vi "Do Request.vi"(7 "Processing In":refnum<class "Processing.lvclass">, 11 "HTTPCmdController in":refnum<class "HTTPCmdController.lvclass">) -> (0 "error out":errorcluster, 5 "Processing":refnum<class "Processing.lvclass">)   [LabVIEW 2020, in "Volatus.lvlib" / "HTTPCmdController.lvclass"]
doc: "A controller's main job is to respond to a request by generating a response. The response value must be specified by calling Set Response.vi on the Processing class that's passed through the VI otherwise an error will be generated.\n\nThere are several helpers available for common response types:\nGenerating HTML content programmatically - Create Basic Response.vi\nStreaming a file from disk - Create File Response.vi\nRedirecting the user to another URL - Create Redirect Response.vi\n\nFile responses are streamed in chunks and do not load the entire file into memory at once to send in the response which allows serving large files more efficiently."
uses:
  HTTPCmdController.lvclass
  lv-http-server/HTTP Server/Processing/Processing.lvclass
  HTTPCmdController.lvclass/HTTPCmdController.ctl
  Http Cmd Type.ctl
  Volatus.lvlib
  Http Chan Cmd.ctl
  MessageQ/MessageQ.lvclass
  lv-http-util/HTTP Utils/Response/Response.lvclass
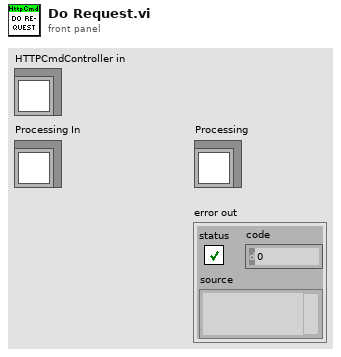
[diagram p1: front panel]
types:
  T1 = typedef "Volatus.lvlib/Http Chan Cmd.ctl" = cluster{"Type":T2, "Channel":string, "Value":dbl}
  T2 = typedef "Volatus.lvlib/Http Cmd Type.ctl" = enum16{"Digital", "Numeric"}
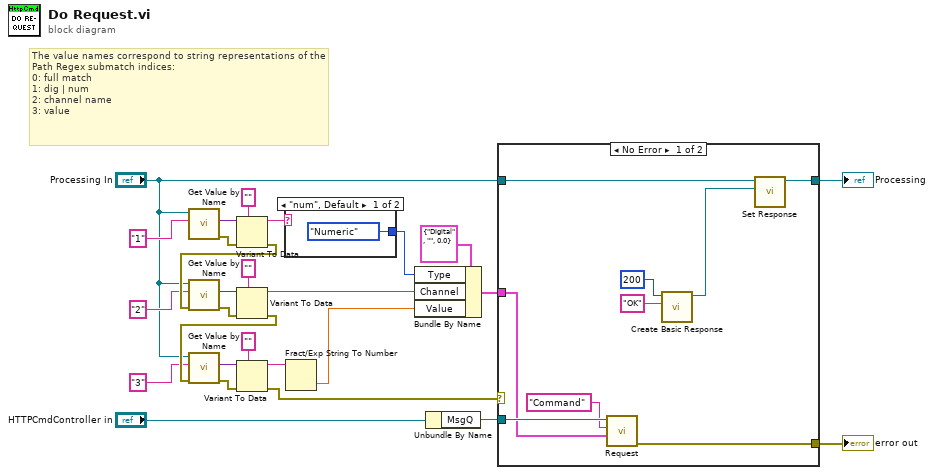
[diagram p0: block diagram]
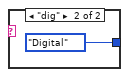
[diagram p3: hidden frame]
diagram:
  # "The value names correspond to string representations of the Path Regex submatch indices:\n0: full match\n1: dig | num\n2: channel name\n3: value"
  n1 = call "Get Value by Name.vi"("Name"="1", "Processing in"="Processing In") -> ("error out"=w10:errorcluster, "Value"=w24:variant)  [unwired: 7 in, 1 out]
  n2 = Variant To Data(error in=w10, type="", Variant=w24) -> (data=w14:string, error out=w27:errorcluster)
  n3 = call "Get Value by Name.vi"("error in (no error)"=w27, "Name"="2", "Processing in"="Processing In") -> ("error out"=w9:errorcluster, "Value"=w21:variant)  [unwired: 6 in, 1 out]
  n4 = Variant To Data(error in=w9, type="", Variant=w21) -> (data=w12:string, error out=w26:errorcluster)
  n5 = call "Get Value by Name.vi"("error in (no error)"=w26, "Name"="3", "Processing in"="Processing In") -> ("error out"=w8:errorcluster, "Value"=w18:variant)  [unwired: 6 in, 1 out]
  n6 = Variant To Data(error in=w8, type="", Variant=w18) -> (data=w16:string, error out=w5:errorcluster)
  n7 = case shown="\"num\", Default" w14 {
    tunnel: [Http_Cmd_Type."Numeric" ("Type") Http_Cmd_Type."Digital" ("Type")] -> w13
    frame "num", Default {
    }
    frame "dig" {
    }
  }
  n8 = Fract/Exp String To Number(string=w16) -> (number=w11:dbl)  [unwired: 3 in, 1 out]
  n9 = Bundle By Name(cluster=T1 {"Type"=enum."Digital", "Channel"="", "Value"=0.0} ("Http Chan Cmd"), "Type"=w13, "Channel"=w12, "Value"=w11) -> (w3:T1)
  n10 = Unbundle By Name("HTTPCmdController in") -> ("MsgQ"=w4:refnum<class "MessageQ.lvclass">)
  n11 = case shown="No Error" w5 {
    selector: w5 -> [_ w39]
    tunnel: "Processing In" -> [w34 w40]
    tunnel: w4 -> [w38 _]
    tunnel: w3 -> [w36 _]
    tunnel: [w35 w39] -> w2
    tunnel: [w31 w40] -> w1
    frame No Error {
      n12 = call "Request.vi"("Data"=w36, "ID"="Command", "MessageQ in"=w38) -> ("error out"=w35:errorcluster)  [unwired: 6 in, 2 out]
      n13 = call "Create Basic Response.vi"("Payload"="OK", "Status Code"=u16 200) -> ("Response out"=w30:refnum<class "Response.lvclass">)  [unwired: 8 in, 1 out]
      n14 = call "Set Response.vi"("Response"=w30, "Processing in"=w34) -> ("Processing out"=w31:refnum<class "Processing.lvclass">)  [unwired: 9 in]
    }
    frame Error {
    }
  }
  "error out" <- w2
  "Processing" <- w1
